vi "Main.vi"(8 "error in":errorcluster, 11 "Settings in":refnum<class "Settings.lvclass">) -> (0 "error out":errorcluster, 3 "Settings out":refnum<class "Settings.lvclass">)   [LabVIEW 2017, in "Settings.lvclass"]
doc: "The <b>Queued Message Handler</b> of the Worker that owns this VI."
uses:
  Settings.lvclass
  <vilib>/Utility/miscctls.llb/LVForegroundBackgroundColorsTypeDef.ctl
  Writable FP Refs.ctl
  Settings.lvclass/Settings.ctl
  Initialization Data.ctl
  Response Cases.ctl
  <vilib>/addons/_Workers/Library/Case Label.ctl
  rqp_Receive Shutdown Data.ctl
  <vilib>/Utility/miscctls.llb/LVRectTypeDef.ctl
  rqp_Load Config Data.ctl
  rsp_Configuration Data.ctl
  Config Data.ctl
  rqp_New Connection Log Message.ctl
  rqp_Client Connected.ctl
  <vilib>/addons/_Workers/Library/Workers.lvlib
panel:
  in  "Cancel":bool
  in  "OK":bool
  in  "Tab Control":enum32{"TCP Server", "Message Log"}(tab)
  out "Server IP Addresses":string
  in  "Server Port":u16=6891
  out "Connection Log":i32(listbox)
  out "Clients Connected":i32
  in  "Max Number of Rows":u16=500 max=5000
  in  "Live Logging Base Folder":path
  in  "Live Logging":bool
  out "Title":string="TCP Server"
  in  "SelectionList":i32(listbox)
  # "Warning: Performance may decrease with a greater number of rows per message log"
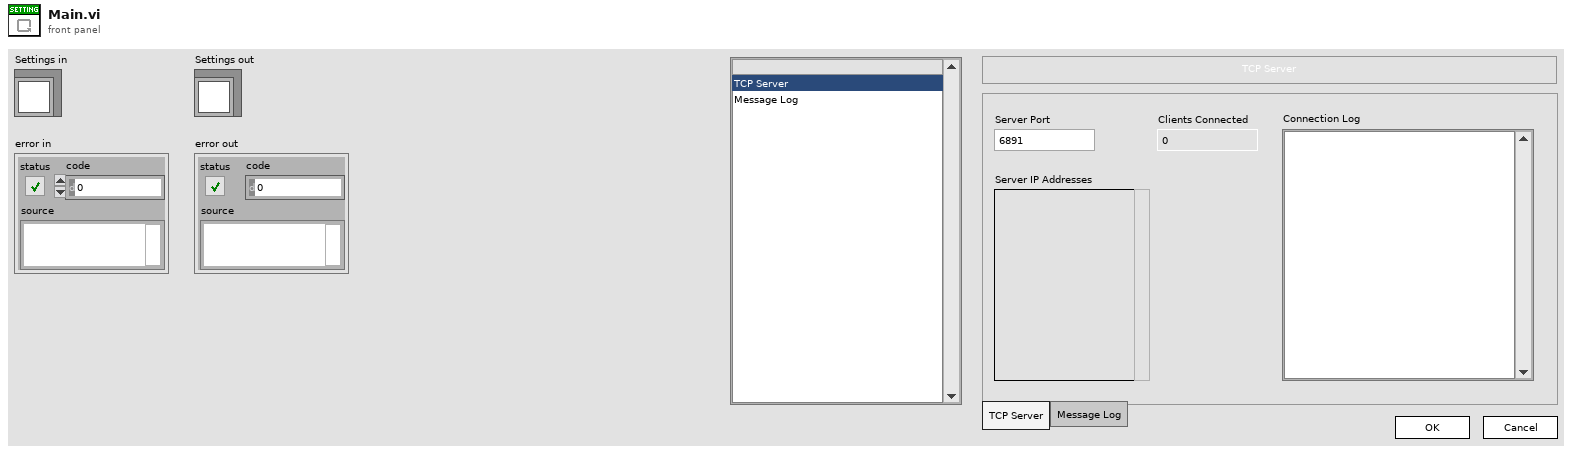
[diagram p1: front panel]
types:
  T1 = typedef "Settings.lvclass/Writable FP Refs.ctl" = cluster{"Server Port":refnum<vi>, "LiveLoggingFolder":refnum<vi>, "LiveLogging":refnum<vi>, "ML.MaxNumRows":refnum<vi>}
  T2 = typedef "LVForegroundBackgroundColorsTypeDef.ctl" = cluster{"Foreground Color":u32, "Background Color":u32}
  T3 = typedef "Settings.lvclass/Initialization Data.ctl" = cluster{"Response Cases":T4}
  T4 = typedef "Settings.lvclass/Response Cases.ctl" = cluster{"Configuration Data":T5, "Shutdown Data Written to File":T5}
  T5 = typedef "Workers.lvlib/Case Label.ctl" = string
  T6 = typedef "Settings.lvclass/rqp_Receive Shutdown Data.ctl" = cluster{"App Manager":cluster{"WinBounds":T7, "FP.State":enum32{"Invalid", "Standard", "Closed", "Hidden", "Minimized", "Maximized"}, "Monitor":u16, "Column Widths":u32[]}, "Message Log":cluster{"Visible Columns":bool[], "Splitter Position":i32, "Column Widths":u32[], "WinBounds":T7, "FP.State":enum32{"Invalid", "Standard", "Closed", "Hidden", "Minimized", "Maximized"}, "Monitor":u16}}
  T7 = typedef "LVRectTypeDef.ctl" = cluster{"Left":i16, "Top":i16, "Right":i16, "Bottom":i16}
  T8 = typedef "Settings.lvclass/rsp_Configuration Data.ctl" = cluster{"Config Data":T9}
  T9 = typedef "Settings.lvclass/Config Data.ctl" = cluster{"DS First Launch":bool, "LogBaseFolder":path, "Live Logging":bool, "Server Port":u16, "Max Number ML Rows":i32, "AM.WinBounds":T7, "AM.FP.State":enum32{"Invalid", "Standard", "Closed", "Hidden", "Minimized", "Maximized"}, "AM.Monitor":u16, "AM.Column Widths":u32[], "ML.Visible Columns":bool[], "ML.Splitter Position":i32, "ML.Column Widths":u32[], "ML.WinBounds":T7, "ML.FP.State":enum32{"Invalid", "Standard", "Closed", "Hidden", "Minimized", "Maximized"}, "ML.Monitor":u16}
  T10 = typedef "Settings.lvclass/rqp_Load Config Data.ctl" = cluster{"String":string}
  T11 = typedef "Settings.lvclass/rqp_New Connection Log Message.ctl" = cluster{"Message":string}
  T12 = typedef "Settings.lvclass/rqp_Client Connected.ctl" = cluster{"Connected":bool}
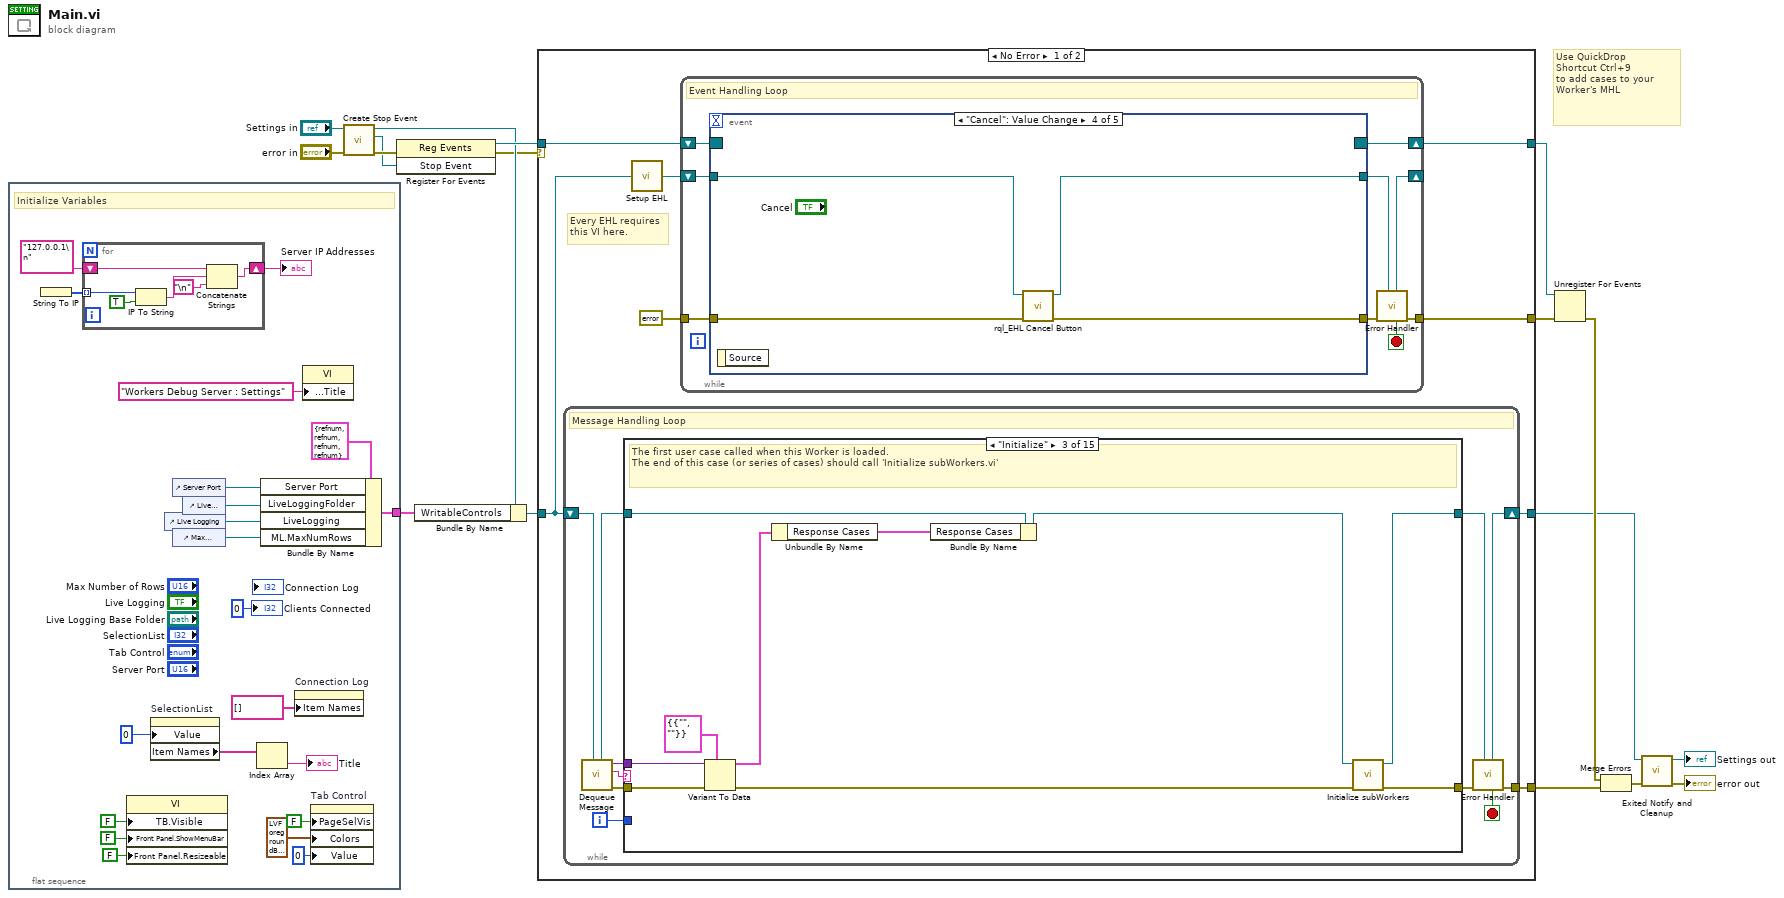
[diagram p0: block diagram]
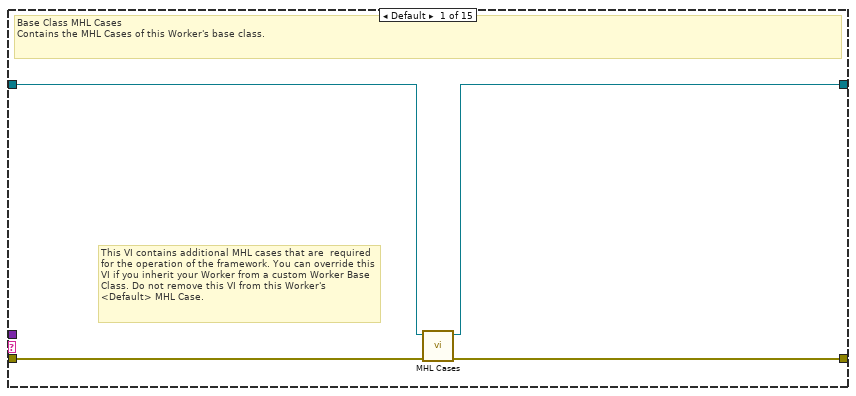
[diagram p2: hidden frame]
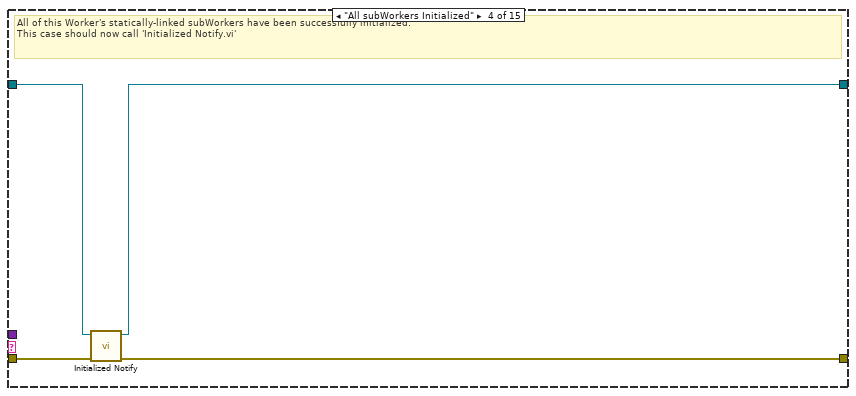
[diagram p4: hidden frame]
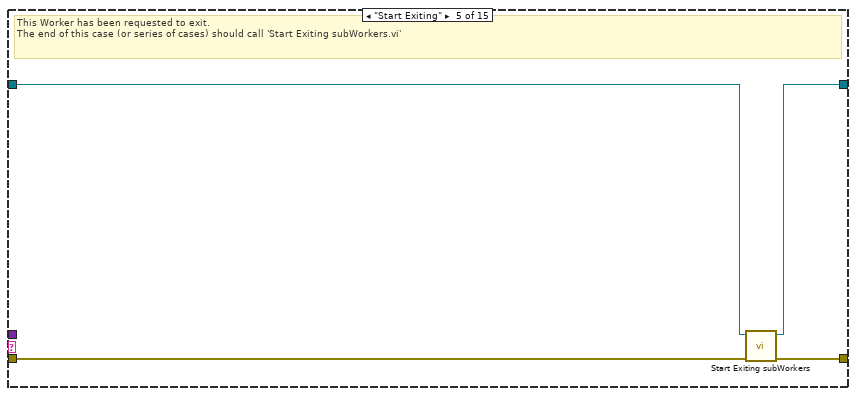
[diagram p5: hidden frame]
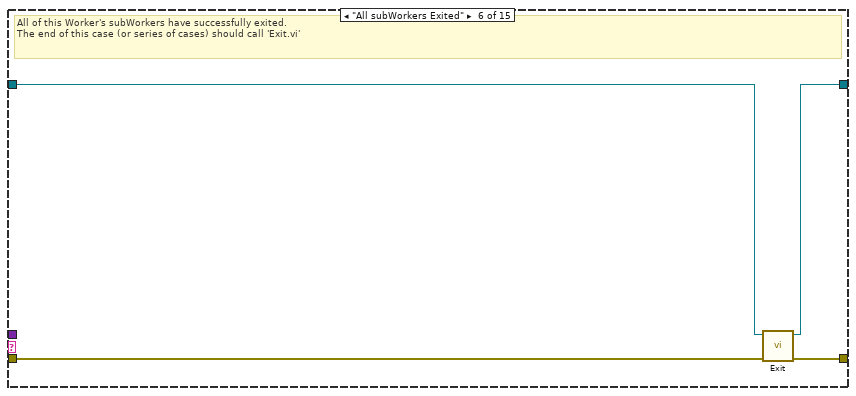
[diagram p6: hidden frame]
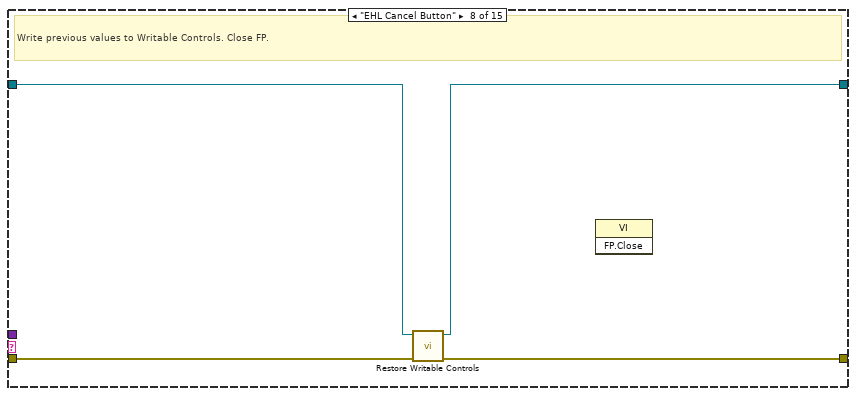
[diagram p8: hidden frame]
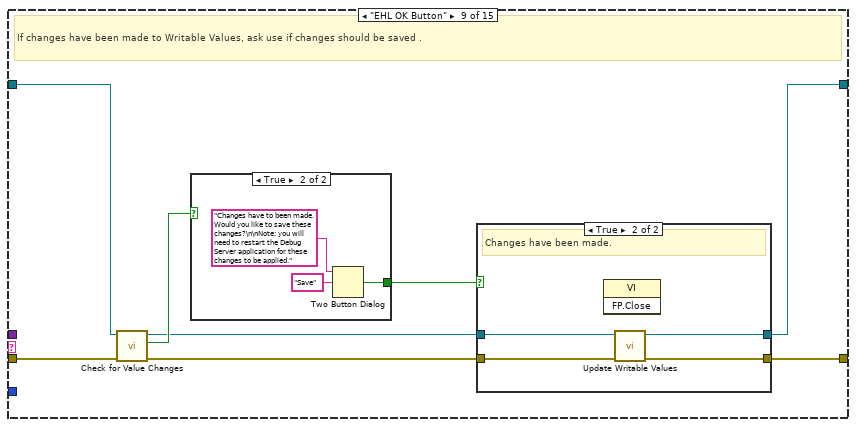
[diagram p9: hidden frame]
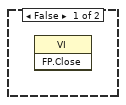
[diagram p11: hidden frame]
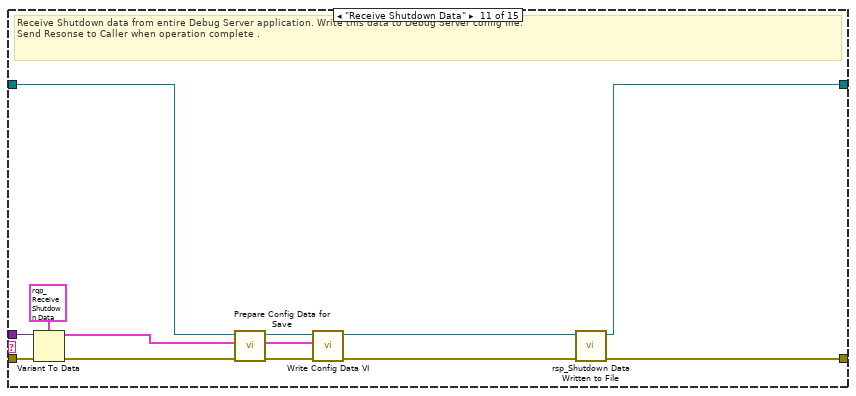
[diagram p13: hidden frame]
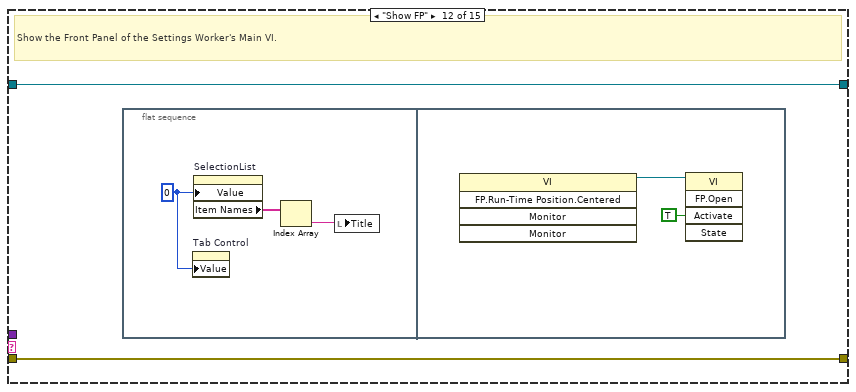
[diagram p14: hidden frame]
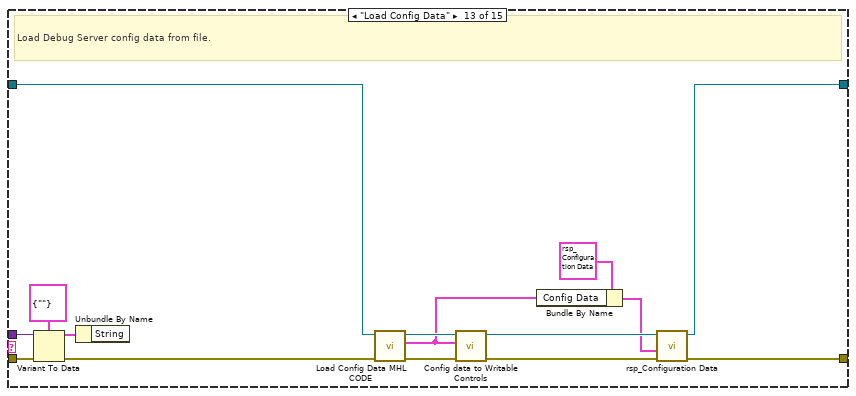
[diagram p15: hidden frame]
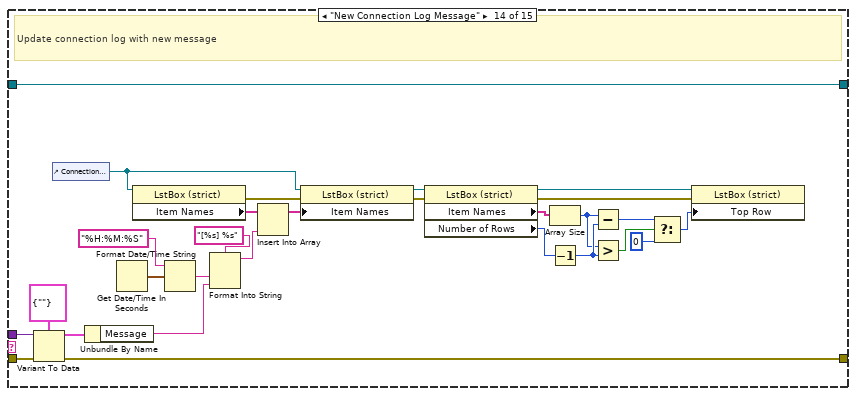
[diagram p16: hidden frame]
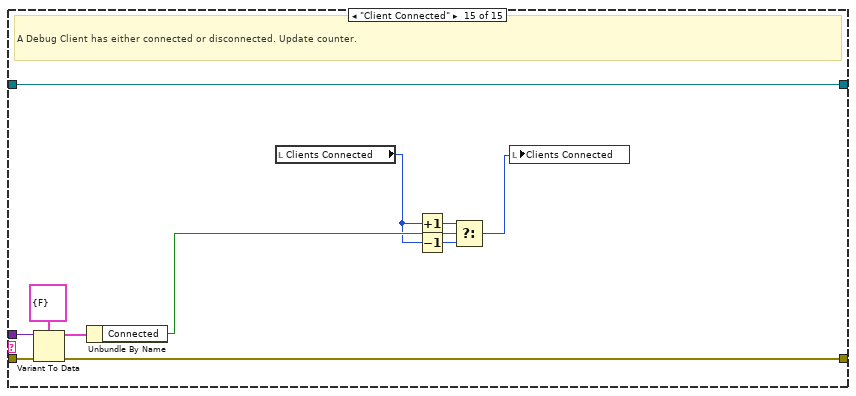
[diagram p17: hidden frame]
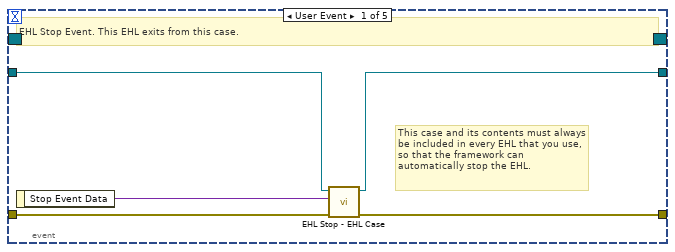
[diagram p18: hidden frame]
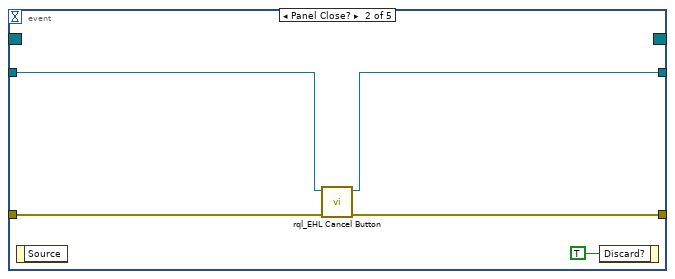
[diagram p19: hidden frame]
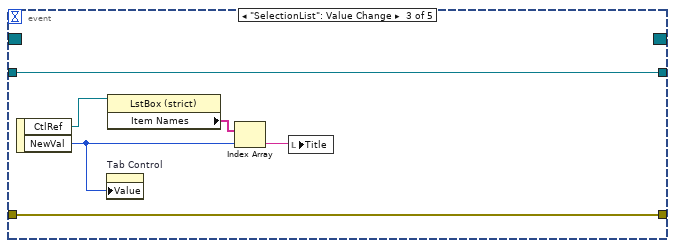
[diagram p20: hidden frame]
diagram:
  # "Use QuickDrop\nShortcut Ctrl+9\nto add cases to your\nWorker's MHL"
  n1 = flat-sequence {
    tunnel: [w38] -> w1
    frame #0 {
      # "Initialize Variables"
      n2 = String To IP() -> (0:w28:u32[])  [unwired: 1 in]
      n3 = for {
        tunnel: w28 -> [w43] mode=indexing
        shift-right: [w39] -> w26
        shift-left: "127.0.0.1\n" -> [w40]
        n4 = IP To String(1:TRUE ("dot notation? (F)"), 2:w43) -> (0:w42:string)
        n5 = Concatenate Strings(w40, w42, "\n") -> (w39:string)
      }
      "Server IP Addresses" <- w26
      n6 = property class="VI"("TB.Visible"=FALSE ("Tool Bar:Visible"), "Front Panel.ShowMenuBar"=FALSE ("Front Panel Window:Show Menu Bar"), "Front Panel.Resizeable"=FALSE ("Front Panel Window:Resizable")) -> ()  [unwired: 2 in, 2 out]
      n7 = property on="SelectionList" class="LstBox (strict)"("Value"=0) -> ("Item Names"=w21:string[])  [unwired: 2 in, 2 out]
      n8 = control-ref of="Live Logging"() -> (w35:refnum<vi>)
      n9 = control-ref of="Server Port"() -> (w37:refnum<vi>)
      n10 = control-ref of="Max Number of Rows"() -> (w31:refnum<vi>)
      n11 = control-ref of="Live Logging Base Folder"() -> (w36:refnum<vi>)
      n12 = Index Array(array=w21) -> (element=→"Title":string)  [unwired: 1 in]
      n13 = Bundle By Name(cluster=T1 {"Server Port"=refnum, "LiveLoggingFolder"=refnum, "LiveLogging"=refnum, "ML.MaxNumRows"=refnum} ("Data"), "Server Port"=w37, "LiveLoggingFolder"=w36, "LiveLogging"=w35, "ML.MaxNumRows"=w31) -> (w38:T1)
      n14 = property on="Connection Log" class="LstBox (strict)"("Item Names"=string[] []) -> ()  [unwired: 2 in, 2 out]
      n15 = property class="VI"("Front Panel.Title"="Workers Debug Server : Settings" ("Front Panel Window:Title")) -> ()  [unwired: 2 in, 2 out]
      n16 = property on="Tab Control" class="TabCtl (strict)"("PageSelVis"=FALSE ("Page Selector Visible"), "Colors"=T2 {"Foreground Color"=16777216, "Background Color"=16777216}, "Value"=0) -> ()  [unwired: 2 in, 2 out]
      "Clients Connected" <- 0 ("Clients Connected")
    }
  }
  n17 = call-dynamic "Create Stop Event.vi"("error in"="error in", "Worker"="Settings in") -> ("error out"=w12:errorcluster, "Stop Event"=w9:refnum<user-event>, "Worker out"=w6:refnum<class "Settings.lvclass">)  [unwired: 7 in]
  n18 = register-events(error in=w12, w9) -> (reference out=w11:refnum<event-registration>, error out=w3:errorcluster)  [unwired: 1 in]
  n19 = Bundle By Name(cluster=w6, "WritableControls"=w1) -> (w2:refnum<class "Settings.lvclass">)
  n20 = case shown="No Error" w3 {
    tunnel: w2 -> [w47 w225]
    tunnel: [w45 w226] -> w10
    tunnel: w11 -> [w52 w227]
    tunnel: [w49 w228] -> w16
    tunnel: [w51 w227] -> w15
    tunnel: [w46 w224] -> w13
    selector: w3 -> [_ w228]
    frame No Error {
      # "Every EHL requires\nthis VI here."
      n21 = while {
        shift-right: [w61] -> w46
        shift-left: w47 -> [w63]
        tunnel: [w62] -> w45
        i -> [w54]
        stop <- w55 stop-if-true
        # "Message Handling Loop"
        n22 = call-dynamic "Dequeue Message.vi"("Worker"=w63) -> ("error out"=w60:errorcluster, "Case out"=w56:string, "Data out"=w53:variant, "Worker out"=w58:refnum<class "Settings.lvclass">)  [unwired: 6 in, 1 out]
        n23 = case "Worker MHL Case Structure (DO NOT CHANGE LABEL NAME)" shown="\"Initialize\"" w56 {
          tunnel: w60 -> [w67 w68 w77 w82 w87 w88 w93 w97 w103 w116 w129 w131 w151 w179 w190]
          tunnel: [w66 w68 w79 w81 w84 w91 w93 w96 w99 w116 w119 w131 w137 w178 w188] -> w59
          tunnel: w58 -> [w65 w69 w76 w83 w86 w89 w92 w95 w104 w115 w123 w130 w140 w174 w189]
          tunnel: [w64 w69 w78 w80 w85 w90 w92 w94 w100 w115 w117 w130 w139 w174 w189] -> w57
          tunnel: w54 -> [_ _ _ _ _ _ _ _ _ _ _ _ _ _ _]
          tunnel: w53 -> [_ _ w74 _ _ _ _ _ _ _ w127 _ w149 w176 w186]
          frame Default {
            # "This VI contains additional MHL cases that are  required for the operation of the framework. You can override this VI if you inherit your Worker from a custom Worker Base Class. Do not remove this VI from this Worker's <Default> MHL Case."
            # "Base Class MHL Cases\nContains the MHL Cases of this Worker's base class."
            n24 = call-dynamic "MHL Cases.vi"("error in"=w67, "Worker in"=w65) -> ("error out"=w66:errorcluster, "Worker out"=w64:refnum<class "Settings.lvclass">)  [unwired: 8 in]
          }
          frame "------------ FRAMEWORK CASES -----------" {
            # "Start of Workers Framework Cases"
          }
          frame "Initialize" {
            # "The first user case called when this Worker is loaded.\nThe end of this case (or series of cases) should call 'Initialize subWorkers.vi'"
            n25 = Variant To Data(error in=w77, type=T3 {"Response Cases"={"Configuration Data"="", "Shutdown Data Written to File"=""}} ("Initialization Data"), Variant=w74) -> (data=w71:T3, error out=w75:errorcluster)
            n26 = Unbundle By Name(w71) -> ("Response Cases"=w70:T4)
            n27 = Bundle By Name(cluster=w76, "Response Cases"=w70) -> (w72:refnum<class "Settings.lvclass">)
            n28 = call-dynamic "Initialize subWorkers.vi"("error in"=w75, "Worker"=w72) -> ("error out"=w79:errorcluster, "dup Worker out"=w78:refnum<class "Settings.lvclass">)  [unwired: 8 in]
          }
          frame "All subWorkers Initialized" {
            # "All of this Worker's statically-linked subWorkers have been successfully initialized.\nThis case should now call 'Initialized Notify.vi'"
            n29 = call-dynamic "Initialized Notify.vi"("error in"=w82, "Worker"=w83) -> ("error out"=w81:errorcluster, "dup Worker out"=w80:refnum<class "Settings.lvclass">)  [unwired: 8 in]
          }
          frame "Start Exiting" {
            # "This Worker has been requested to exit. \nThe end of this case (or series of cases) should call 'Start Exiting subWorkers.vi'"
            n30 = call-dynamic "Start Exiting subWorkers.vi"("error_in"=w87, "Worker"=w86) -> ("error out"=w84:errorcluster, "dup Worker out"=w85:refnum<class "Settings.lvclass">)  [unwired: 8 in]
          }
          frame "All subWorkers Exited" {
            # "All of this Worker's subWorkers have successfully exited. \nThe end of this case (or series of cases) should call 'Exit.vi'"
            n31 = call-dynamic "Exit.vi"("error_in"=w88, "Worker"=w89) -> ("error out"=w91:errorcluster, "dup Worker out"=w90:refnum<class "Settings.lvclass">)  [unwired: 8 in]
          }
          frame "------------- LOCAL API CASES -------------" {
            # "Start of Workers Local API Cases"
          }
          frame "EHL Cancel Button" {
            # "Write previous values to Writable Controls. Close FP."
            n32 = call "Restore Writable Controls.vi"("error in (no error)"=w97, "Settings in"=w95) -> ("error out"=w96:errorcluster, "Settings out"=w94:refnum<class "Settings.lvclass">)  [unwired: 8 in]
            n33 = invoke class="VI" method="FP.Close"() -> ()  [unwired: 3 in, 3 out]
          }
          frame "EHL OK Button" {
            # "If changes have been made to Writable Values, ask use if changes should be saved ."
            n34 = call "Check for Value Changes.vi"("error in (no error)"=w103, "Settings in"=w104) -> ("error out"=w105:errorcluster, "Changes have been made"=w102:bool, "Settings out"=w101:refnum<class "Settings.lvclass">)  [unwired: 7 in]
            n35 = case shown="True" w102 {
              tunnel: [_ w112] -> w98
              frame False {
                n36 = invoke class="VI" method="FP.Close"() -> ()  [unwired: 3 in, 3 out]
              }
              frame True {
                n37 = Two Button Dialog(message="Changes have to been made. Would you like to save these changes?\n\nNote: you will need to restart the Debug Server application for these changes to be applied.", 2:"Save" ("T button name (\"OK\")")) -> (T button?=w112:bool)  [unwired: 1 in]
              }
            }
            n38 = case shown="True" w98 {
              tunnel: w105 -> [w107 w111]
              tunnel: w101 -> [w106 w110]
              tunnel: [w106 w109] -> w100
              tunnel: [w107 w108] -> w99
              frame False {
                # "No changes made or User cancelled the operation."
              }
              frame True {
                # "Changes have been made."
                n39 = invoke class="VI" method="FP.Close"() -> ()  [unwired: 3 in, 3 out]
                n40 = call "Update Writable Values.vi"("error in (no error)"=w111, "Settings in"=w110) -> ("error out"=w108:errorcluster, "Settings out"=w109:refnum<class "Settings.lvclass">)  [unwired: 8 in]
              }
            }
          }
          frame "------------- PUBLIC API CASES -------------" {
            # "Start of Workers Public API Cases"
          }
          frame "Receive Shutdown Data" {
            # "Receive Shutdown data from entire Debug Server application. Write this data to Debug Server config file.\nSend Resonse to Caller when operation complete ."
            n41 = Variant To Data(error in=w129, type=T6 {"App Manager"={"WinBounds"={"Left"=0, "Top"=0, "Right"=0, "Bottom"=0}, "FP.State"=enum."Invalid", "Monitor"=0, "Column Widths"=[]}, "Message Log"={"Visible Columns"=[], "Splitter Position"=0, "Column Widths"=[], "WinBounds"={"Left"=0, "Top"=0, "Right"=0, "Bottom"=0}, "FP.State"=enum."Invalid", "Monitor"=0}} ("Data"), Variant=w127) -> (data=w120:T6, error out=w126:errorcluster)
            n42 = call "Prepare Config Data for Save.vi"("error in (no error)"=w126, "Shutdown Data"=w120, "Settings in"=w123) -> ("error out"=w124:errorcluster, "Config Data"=w121:T9, "Settings out"=w122:refnum<class "Settings.lvclass">)  [unwired: 6 in]
            n43 = call "Write Config Data VI.vi"("error in (no error)"=w124, "Config Data"=w121, "Settings in"=w122) -> ("error out"=w125:errorcluster, "Settings out"=w118:refnum<class "Settings.lvclass">)  [unwired: 7 in]
            n44 = call "rsp_Shutdown Data Written to File.vi"("error in"=w125, "Settings in"=w118) -> ("error out"=w119:errorcluster, "dup Settings out"=w117:refnum<class "Settings.lvclass">)  [unwired: 8 in]
          }
          frame "Show FP" {
            # "Show the Front Panel of the Settings Worker's Main VI."
            n45 = flat-sequence {
              frame #0 {
                w134 = 0
                n46 = property on="Tab Control" class="TabCtl (strict)"("Value"=w134) -> ()  [unwired: 2 in, 2 out]
                n47 = property on="SelectionList" class="LstBox (strict)"("Value"=w134) -> ("Item Names"=w132:string[])  [unwired: 2 in, 2 out]
                n48 = Index Array(array=w132) -> (element=w133:string)  [unwired: 1 in]
                n49 = local write "Title"(w133) -> ()
              }
              frame #1 {
                n50 = invoke class="VI" method="FP.Run-Time Position.Centered"() -> (reference out=w135:refnum<vi>)  [unwired: 5 in, 4 out]
                n51 = invoke class="VI" method="FP.Open"(reference=w135, "Activate"=TRUE ("Activate?")) -> ()  [unwired: 3 in, 5 out]
              }
            }
          }
          frame "Load Config Data" {
            # "Load Debug Server config data from file."
            n52 = Variant To Data(error in=w151, type=T10 {"String"=""} ("Data"), Variant=w149) -> (data=w148:T10, error out=w138:errorcluster)
            n53 = Unbundle By Name(w148) -> ()  [unwired: 1 out]
            n54 = call "Load Config Data MHL CODE.vi"("error in (no error)"=w138, "Settings in"=w140) -> ("error out"=w147:errorcluster, "Config Data"=w144:T9, "Settings out"=w146:refnum<class "Settings.lvclass">)  [unwired: 7 in]
            n55 = call "Config data to Writable Controls.vi"("error in (no error)"=w147, "Config Data"=w144, "Settings in"=w146) -> ("error out"=w145:errorcluster, "Settings out"=w142:refnum<class "Settings.lvclass">)  [unwired: 7 in]
            n56 = Bundle By Name(cluster=T8 {"Config Data"={"DS First Launch"=FALSE, "LogBaseFolder"=path "", "Live Logging"=FALSE, "Server Port"=0, "Max Number ML Rows"=0, "AM.WinBounds"={"Left"=0, "Top"=0, "Right"=0, "Bottom"=0}, "AM.FP.State"=enum."Invalid", "AM.Monitor"=0, "AM.Column Widths"=[], "ML.Visible Columns"=[], "ML.Splitter Position"=0, "ML.Column Widths"=[], "ML.WinBounds"={"Left"=0, "Top"=0, "Right"=0, "Bottom"=0}, "ML.FP.State"=enum."Invalid", "ML.Monitor"=0}} ("Data"), "Config Data"=w144) -> (w141:T8)
            n57 = call "rsp_Configuration Data.vi"("error in"=w145, "Data in"=w141, "Settings in"=w142) -> ("error out"=w137:errorcluster, "dup Settings out"=w139:refnum<class "Settings.lvclass">)  [unwired: 7 in]
          }
          frame "New Connection Log Message" {
            # "Update connection log with new message"
            n58 = Variant To Data(error in=w179, type=T11 {"Message"=""} ("Data"), Variant=w176) -> (data=w175:T11, error out=w178:errorcluster)
            n59 = control-ref of="Connection Log"() -> (w173:refnum<vi>)
            n60 = Unbundle By Name(w175) -> ("Message"=w152:string)
            n61 = Get Date/Time In Seconds() -> (seconds since 1Jan1904=w159:timestamp)
            n62 = property class="LstBox (strict)"(reference=w173) -> (error out=w156:errorcluster, "Item Names"=w157:string[])  [unwired: 1 in, 1 out]
            n63 = Format Date/Time String(time format string (%c)="%H:%M:%S", seconds (now)=w159) -> (date/time string=w160:string)  [unwired: 1 out]
            n64 = Format Into String(format string="[%s] %s", w160, w152) -> (resulting string=w161:string)  [unwired: 2 in, 1 out]
            n65 = Insert Into Array(array=w157, new element=w161) -> (w158:string[])  [unwired: 1 in]
            n66 = property class="LstBox (strict)"(reference=w173, error in=w156, "Item Names"=w158) -> (reference out=w169:refnum<vi>, error out=w171:errorcluster)
            n67 = property class="LstBox (strict)"(reference=w169, error in=w171) -> (reference out=w170:refnum<vi>, error out=w172:errorcluster, "Item Names"=w165:string[], "Number of Rows"=w166:u32)
            n68 = Array Size(array=w165) -> (size(s)=w163:i32)
            n69 = Decrement(x=w166) -> (x-1=w168:u32)
            n70 = Subtract(x=w163, y=w168) -> (x-y=w164:u32)
            n71 = Greater?(x=w163, y=w168) -> (0:w162:bool)
            n72 = Select(t=w164, s=w162, f=u32 0) -> (s? t:f=w167:u32)
            n73 = property class="LstBox (strict)"(reference=w170, error in=w172, "Top Row"=w167) -> ()  [unwired: 2 out]
          }
          frame "Client Connected" {
            # "A Debug Client has either connected or disconnected. Update counter."
            n74 = Variant To Data(error in=w190, type=T12 {"Connected"=FALSE} ("Data"), Variant=w186) -> (data=w185:T12, error out=w188:errorcluster)
            n75 = Unbundle By Name(w185) -> ("Connected"=w183:bool)
            n76 = local read "Clients Connected"() -> (w181:i32)
            n77 = Increment(x=w181) -> (x+1=w182:i32)
            n78 = Decrement(x=w181) -> (x-1=w184:i32)
            n79 = Select(t=w182, s=w183, f=w184) -> (s? t:f=w180:i32)
            n80 = local write "Clients Connected"(w180) -> ()
          }
        }
        n81 = call-dynamic "Error Handler.vi"("Worker"=w57, "error_in"=w59) -> ("error out"=w62:errorcluster, "Stop Loop"=w55:bool, "Worker out"=w61:refnum<class "Settings.lvclass">)  [unwired: 7 in]
      }
      n82 = call-dynamic "Setup EHL.vi"("Worker"=w47) -> ("Worker out"=w48:refnum<class "Settings.lvclass">)  [unwired: 14 in]
      n83 = while "Event Handling Loop" {
        shift-right: [w199] -> w51
        shift-left: w52 -> [w198]
        tunnel: [w194] -> w49
        tunnel: errorcluster {"status"=FALSE, "code"=0, "source"=""} ("error constant") -> [w196]
        shift-right: [w192] -> _
        shift-left: w48 -> [w197]
        stop <- w191 stop-if-true
        # "Event Handling Loop"
        n84 = event shown="[3] \"Cancel\": Value Change" {
          selector: w198 -> [_ _ _ _ _]
          dyn-events: [_ _ _ _ _] -> w199
          timeout: _ -> [_ _ _ _ _]
          tunnel: [w203 w207 w215 w218 w222] -> w195
          tunnel: w196 -> [w204 w208 w215 w219 w223]
          tunnel: w197 -> [w202 w206 w214 w217 w221]
          tunnel: [w201 w205 w214 w216 w220] -> w193
          event User Event {
            # "This case and its contents must always be included in every EHL that you use, so that the framework can automatically stop the EHL."
            # "EHL Stop Event. This EHL exits from this case."
            n85 = event-data() -> ("Stop Event Data"=w200:variant)  [unwired: 1 in]
            n86 = call-dynamic "EHL Stop - EHL Case.vi"("error in"=w204, "Stop Event Data"=w200, "Worker"=w202) -> ("error out"=w203:errorcluster, "Worker out"=w201:refnum<class "Settings.lvclass">)  [unwired: 7 in]
          }
          event Panel Close? {
            n87 = event-data() -> ()  [unwired: 1 in, 1 out]
            n88 = call "rql_EHL Cancel Button.vi"("error in"=w208, "Settings in"=w206) -> ("error out"=w207:errorcluster, "dup Settings out"=w205:refnum<class "Settings.lvclass">)  [unwired: 8 in]
            n89 = event-data("Discard?"=TRUE) -> ()  [unwired: 1 in, 1 out]
          }
          event "SelectionList": Value Change {
            n90 = event-data() -> ("CtlRef"=w213:refnum<vi>, "NewVal"=w211:i32)  [unwired: 1 in]
            n91 = property on="Tab Control" class="TabCtl (strict)"("Value"=w211) -> ()  [unwired: 2 in, 2 out]
            n92 = property class="LstBox (strict)"(reference=w213) -> ("Item Names"=w212:string[])  [unwired: 1 in, 2 out]
            n93 = Index Array(array=w212, index=w211) -> (element=w210:string)
            n94 = local write "Title"(w210) -> ()
          }
          event "Cancel": Value Change {
            n95 = event-data() -> ()  [unwired: 1 in, 1 out]
            n96 = call "rql_EHL Cancel Button.vi"("error in"=w219, "Settings in"=w217) -> ("error out"=w218:errorcluster, "dup Settings out"=w216:refnum<class "Settings.lvclass">)  [unwired: 8 in]
          }
          event "OK": Value Change {
            n97 = event-data() -> ()  [unwired: 1 in, 1 out]
            n98 = call "rql_EHL OK Button.vi"("error in"=w223, "Settings in"=w221) -> ("error out"=w222:errorcluster, "dup Settings out"=w220:refnum<class "Settings.lvclass">)  [unwired: 8 in]
          }
        }
        n99 = call-dynamic "Error Handler.vi"("Worker"=w193, "error_in"=w195) -> ("error out"=w194:errorcluster, "Stop Loop"=w191:bool, "Worker out"=w192:refnum<class "Settings.lvclass">)  [unwired: 7 in]
      }
    }
    frame Error {
      n100 = call-dynamic "Error Handler.vi"("Worker"=w225, "error_in"=w228) -> ("error out"=w226:errorcluster, "Worker out"=w224:refnum<class "Settings.lvclass">)  [unwired: 7 in, 1 out]
    }
  }
  n101 = Unregister For Events(event registration refnum=w15, error in=w16) -> (error out=w17:errorcluster)
  n102 = Merge Errors(w17, w10) -> (w14:errorcluster)
  n103 = call-dynamic "Exited Notify and Cleanup.vi"("error_in"=w14, "Worker"=w13) -> ("error out"=→"error out":errorcluster, "dup Worker out"=→"Settings out":refnum<class "Settings.lvclass">)  [unwired: 8 in]
